vi "24BitTo3U8.vi"(8 "2-Bit Suffix":u8 format="%02b", 9 "4-Bit Prefix":u8=16 format="%04b", 11 "18-Bit":u32=16 format="%018b") -> (3 "3 U8":u8[](array[numeric]) format="%08b")   [LabVIEW 2014]
panel:
  out "U8 2":u8 format="%08b"
  out "U8":u8 format="%08b"
  out "i":i32
  out "executions":i32
  in  "planned executions":i32
  out "U32 5":i32 format="%032b"
  in  "U32 4":i32 format="%032b"
  out "PortOut 2":bool
  out "PortOut":bool
  out "PortSelectOut":u8 format="%08b"
  in  "PortSelect":u8 format="%08b"
  out "U32 3":u32 format="%032b"
  in  "U32 2":u32 format="%0d"
  out "array w/ subset deleted":u8[](array[numeric]) format="%08b"
  in  "U32":u32 format="%032b"
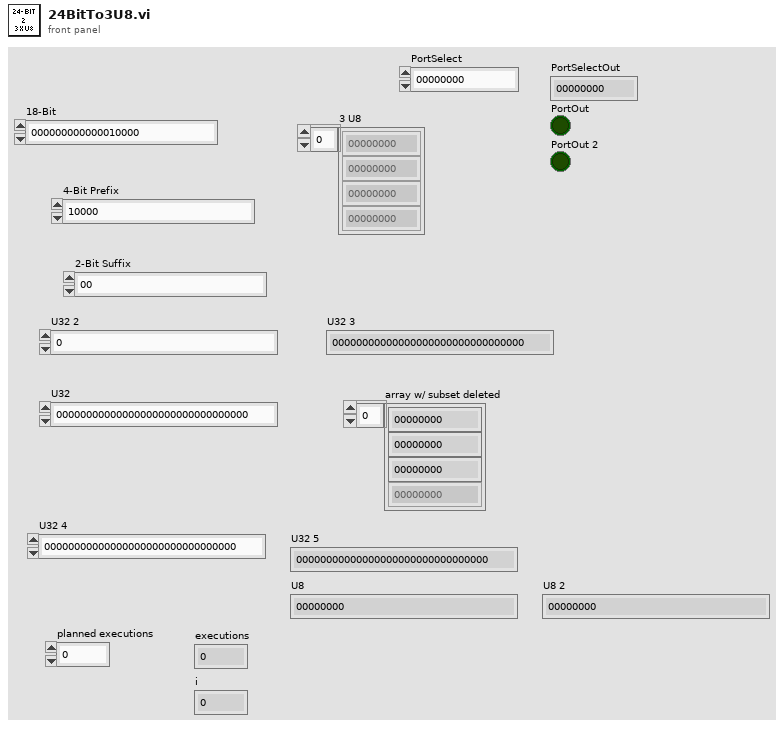
[diagram p1: front panel]
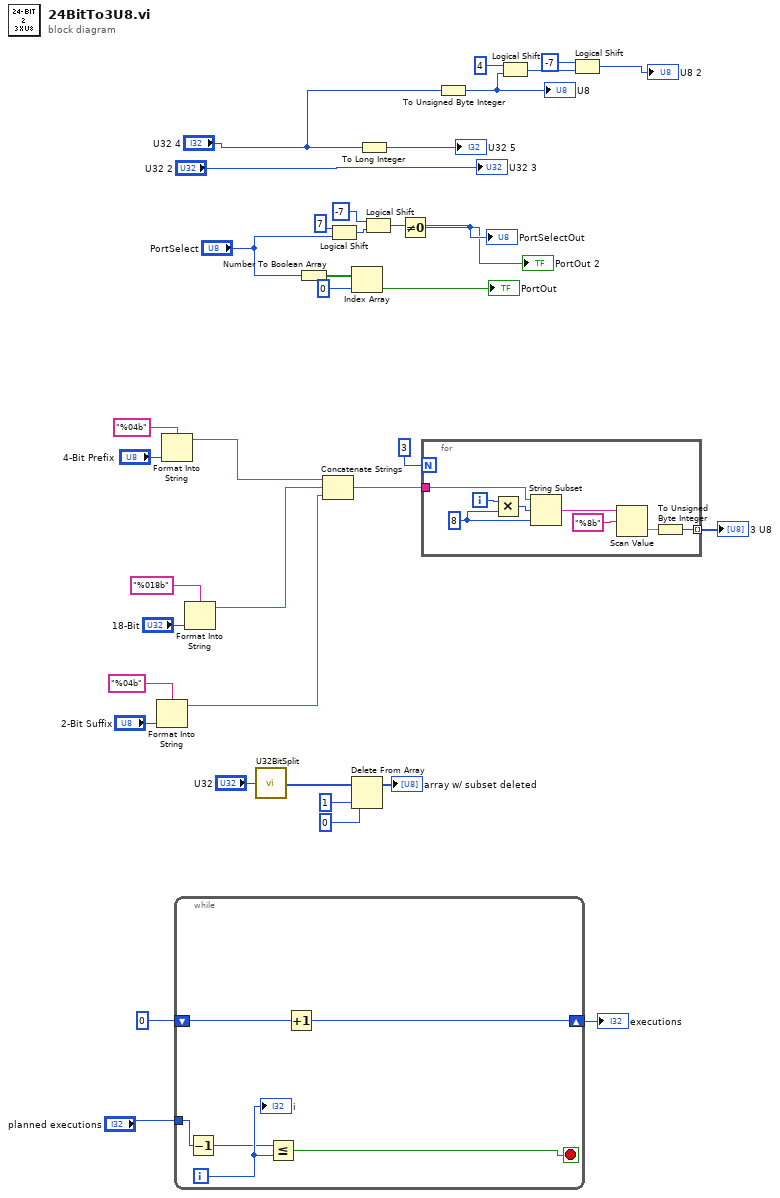
[diagram p0: block diagram]
diagram:
  n1 = Format Into String(format string="%04b", "2-Bit Suffix") -> (resulting string=w26:string)  [unwired: 2 in, 1 out]
  n2 = Format Into String(format string="%04b", "4-Bit Prefix") -> (resulting string=w31:string)  [unwired: 2 in, 1 out]
  n3 = while {
    shift-right: [w42] -> w8
    shift-left: 0 ("Numeric") -> [w43]
    tunnel: "planned executions" -> [w40]
    i -> [w39]
    stop <- w41 stop-if-true
    n4 = Decrement(x=w40) -> (x-1=w38:i32)
    n5 = Less Or Equal?(x=w38, y=w39) -> (x <= y?=w41:bool)
    n6 = Increment(x=w43) -> (x+1=w42:i32)
    "i" <- w39
  }
  "executions" <- w8
  n7 = Format Into String(format string="%018b", "18-Bit") -> (resulting string=w30:string)  [unwired: 2 in, 1 out]
  n8 = call "U32BitSplit.vi"("U32"="U32") -> ("U8 Array"=w24:u8[])
  n9 = Number To Boolean Array(number="PortSelect") -> (Boolean array=w19:bool[])
  n10 = Concatenate Strings(w31, w30, w26) -> (w29:string)
  n11 = Logical Shift(y=i16 7, x="PortSelect") -> (x << y=w14:u8)
  n12 = Index Array(array=w19, index=0) -> (element=→"PortOut":bool)
  n13 = Delete From Array(array=w24, length=1, index=0) -> (array with subset deleted=→"array w/ subset deleted":u8[])  [unwired: 1 out]
  n14 = To Long Integer(number="U32 4") -> (32bit integer=→"U32 5":i32)
  n15 = Logical Shift(y=i16 -7, x=w14) -> (x << y=w12:u8)
  "PortSelectOut" <- w12
  n16 = Not Equal To 0?(x=w12) -> (x != 0?=→"PortOut 2":bool)
  n17 = for {
    N: 3 -> [_]
    tunnel: w29 -> [w51]
    tunnel: [w44] -> w34 mode=indexing
    i -> [w48]
    w46 = 8 ("y")
    n18 = Multiply(x=w48, y=w46) -> (x*y=w47:i32)
    n19 = String Subset(string=w51, offset (0)=w47, length (rest)=w46) -> (substring=w50:string)
    n20 = Scan Value(string=w50, format string="%8b") -> (value=w45:dbl)  [unwired: 1 in, 1 out]
    n21 = To Unsigned Byte Integer(number=w45) -> (unsigned 8bit integer=w44:u8)
  }
  "3 U8" <- w34
  n22 = To Unsigned Byte Integer(number="U32 4") -> (unsigned 8bit integer=w5:u8)
  "U8" <- w5
  n23 = Logical Shift(y=i8 4, x=w5) -> (x << y=w3:u8)
  n24 = Logical Shift(y=i8 -7, x=w3) -> (x << y=→"U8 2":u8)
  "U32 3" <- "U32 2"
